vi "FTW-Inbox-Core-Configuration.vi"(5 "Inbox Configuration":string="{\n  \"MaxMessageSize\": 100000,\n  \"AdditionalServiceEndpoints\":\n  {\n    \"Primary\": \"tcp://127.0.0.1:*\",\n    \"RemoteClients\": \"ws://*:*\"\n  },\n  \"MessageRoutingRules\":\n  {\n    \"FTW-PoisonPill\":\n    {\n      \"Accept\": true,\n      \"Reject\": false\n    },\n    \"FTW-ActorStatus\":\n    {\n      \"Accept\": true,\n      \"Reject\": false,\n      \"BusyTimeout\": 100,\n      \"ResponseIncludesIdentity\": true,\n      \"ResponseIncludesTimestamp\": true,\n      \"ResponseIncludesRelativeTimer\": true\n    },\n    \"Default\":\n    {\n      \"Accept\": false,\n      \"Reject\": false,\n      \"BusyTimeout\": -1,\n      \"ResponseIncludesIdentity\": true,\n      \"ResponseIncludesTimestamp\": true,\n      \"ResponseIncludesRelativeTimer\": true\n    }\n  }\n}", 11 "error in":errorcluster) -> (4 "Message Routing Rules":T1[](array[typedef]) {"SendTimeout" format="%dmsec"; "BusyTimeout" format="%dmsec"}, 6 "Additional Endpoint Addresses":string[](array[string]), 8 "Receive Message Size Limit":i32=1000 format="%_4pbytes", 10 "AdditionalServiceEndpoints":string, 15 "error out":errorcluster)   [LabVIEW 2015]
uses:
  FTW-Inbox-Core-RoutingRule.ctl
  lib/FTW-KernelFilepath.vi
  error/FTW-ERR-ThrowError.vi
  json/core/FTW-JSON-Core-EncodingFlags.vi
  reflection/FTW-Reflection-Type.vi
  codegen/xnode/json/fetch/FTW-JSON-Core-GetFlattenedValue.vi
  error/FTW-ERR-NoErrorConstant.vi
  codegen/xnode/FTW-JSON-Fetch.xnode
panel:
  # "Inputs"
  # "Outputs"
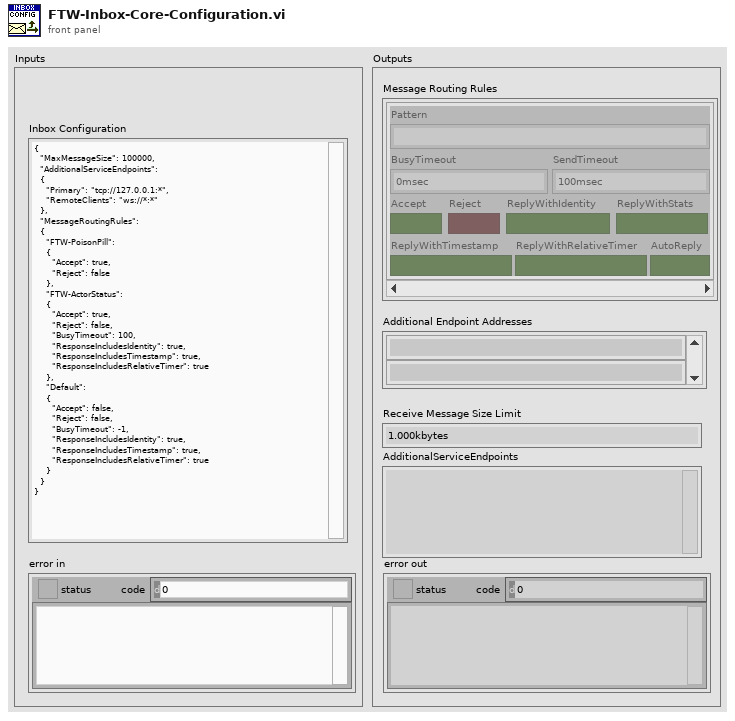
[diagram p1: front panel]
types:
  T1 = typedef "FTW-Inbox-Core-RoutingRule.ctl" = cluster{"Pattern":string, "BusyTimeout":i32, "SendTimeout":i32, "Accept":bool, "Reject":bool, "ReplyWithIdentity":bool, "ReplyWithStats":bool, "ReplyWithTimestamp":bool, "ReplyWithRelativeTimer":bool, "AutoReply":bool}
  T2 = cluster{"MaxMessageSize":i32, "MessageRoutingRules":string, "AdditionalServiceEndpoints":string, "MessageRoutingRules":cluster{"Default":cluster{"Pattern":string, "BusyTimeout":i32, "SendTimeout":i32, "Accept":bool, "Reject":bool, "ReplyWithIdentity":bool, "ReplyWithStatistics":bool, "ReplyWithTimestamp":bool, "ReplyWithRelativeTimer":bool, "AutoReply":bool}, "FTW-PoisonPill":cluster{"Pattern":string, "BusyTimeout":i32, "SendTimeout":i32, "Accept":bool, "Reject":bool, "ReplyWithIdentity":bool, "ReplyWithStatistics":bool, "ReplyWithTimestamp":bool, "ReplyWithRelativeTimer":bool, "AutoReply":bool}, "FTW-ActorStatus":cluster{"Pattern":string, "BusyTimeout":i32, "SendTimeout":i32, "Accept":bool, "Reject":bool, "ReplyWithIdentity":bool, "ReplyWithStatistics":bool, "ReplyWithTimestamp":bool, "ReplyWithRelativeTimer":bool, "AutoReply":bool}}}
  T3 = cluster{"Pattern":string, "BusyTimeout":i32, "SendTimeout":i32, "Accept":bool, "Reject":bool, "ReplyWithIdentity":bool, "ReplyWithStatistics":bool, "ReplyWithTimestamp":bool, "ReplyWithRelativeTimer":bool, "AutoReply":bool}
  T4 = typedef "FTW-Type-JSON.ctl" = refnum<data-value>
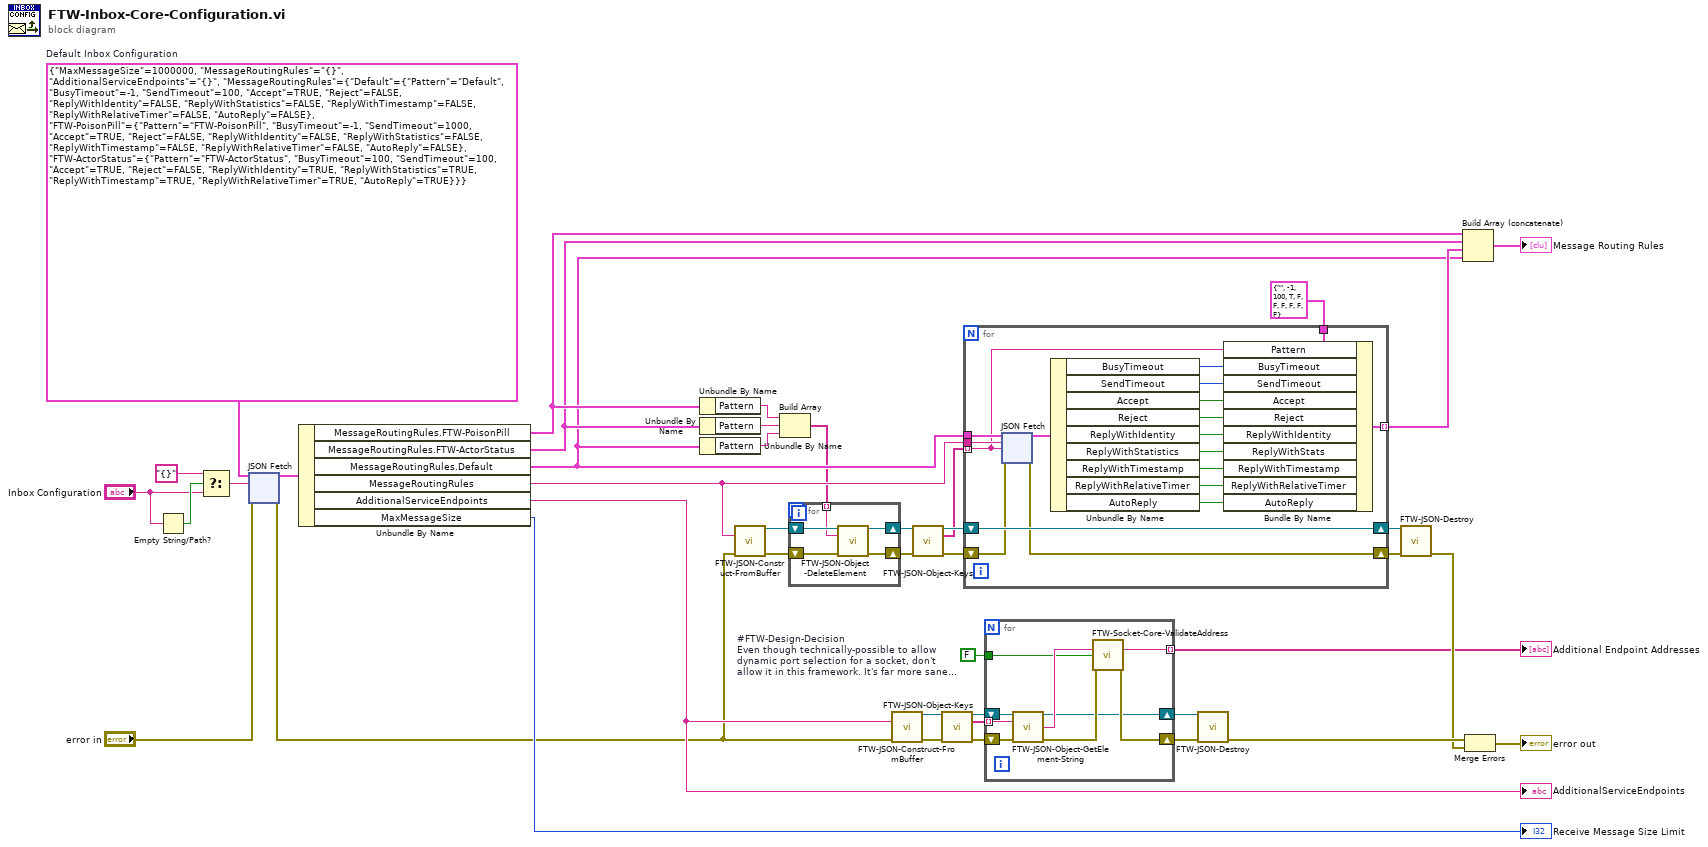
[diagram p0: block diagram]
diagram:
  w17 = FALSE  # #FTW-Design-Decision Even though technically-possible to allow dynamic port selection for a socket, don't allow it in this framework. It's far more sane to fix static addresses agreed upon by all nodes in the system.
  w5 = T2 {"MaxMessageSize"=1000000, "MessageRoutingRules"="{}", "AdditionalServiceEndpoints"="{}", "MessageRoutingRules"={"Default"={"Pattern"="Default", "BusyTimeout"=-1, "SendTimeout"=100, "Accept"=TRUE, "Reject"=FALSE, "ReplyWithIdentity"=FALSE, "ReplyWithStatistics"=FALSE, "ReplyWithTimestamp"=FALSE, "ReplyWithRelativeTimer"=FALSE, "AutoReply"=FALSE}, "FTW-PoisonPill"={"Pattern"="FTW-PoisonPill", "BusyTimeout"=-1, "SendTimeout"=1000, "Accept"=TRUE, "Reject"=FALSE, "ReplyWithIdentity"=FALSE, "ReplyWithStatistics"=FALSE, "ReplyWithTimestamp"=FALSE, "ReplyWithRelativeTimer"=FALSE, "AutoReply"=FALSE}, "FTW-ActorStatus"={"Pattern"="FTW-ActorStatus", "BusyTimeout"=100, "SendTimeout"=100, "Accept"=TRUE, "Reject"=FALSE, "ReplyWithIdentity"=TRUE, "ReplyWithStatistics"=TRUE, "ReplyWithTimestamp"=TRUE, "ReplyWithRelativeTimer"=TRUE, "AutoReply"=TRUE}}}  # Default Inbox Configuration
  n1 = Empty String/Path?(string/path="Inbox Configuration") -> (empty?=w8:bool)
  n2 = Select(t="{}", s=w8, f="Inbox Configuration") -> (s? t:f=w3:string)
  n3 = xnode "JSON Fetch"("Type and Defaults"=w5, "JSON String"=w3, "error in"="error in") -> ("Values"=w4:T2, "error out"=w1:errorcluster)  [unwired: 1 in]
  n4 = Unbundle By Name(w4) -> ("MessageRoutingRules.FTW-PoisonPill"=w15:T3, "MessageRoutingRules.FTW-ActorStatus"=w14:T3, "MessageRoutingRules.Default"=w13:T3, "MessageRoutingRules"=w16:string, "AdditionalServiceEndpoints"=w42:string, "MaxMessageSize"=→"Receive Message Size Limit":i32)
  "AdditionalServiceEndpoints" <- w42
  n5 = Unbundle By Name(w15) -> ("Pattern"=w12:string)
  n6 = Unbundle By Name(w14) -> ("Pattern"=w11:string)
  n7 = Unbundle By Name(w13) -> ("Pattern"=w10:string)
  n8 = call "FTW-JSON-Construct-FromBuffer.vi"("JSON String (UTF-8)"=w16, "error in"=w1) -> ("JSON"=w23:T4, "error out"=w21:errorcluster)  [unwired: 12 in]
  n9 = Build Array(w12, w11, w10) -> (w9:string[])
  n10 = for {
    shift-right: [w46] -> w22
    shift-left: w23 -> [w47]
    shift-right: [w44] -> w20
    shift-left: w21 -> [w45]
    tunnel: w9 -> [w43] mode=indexing
    n11 = call "FTW-JSON-Object-DeleteElement.vi"("JSON"=w47, "Key"=w43, "error in"=w45) -> ("JSON out"=w46:T4, "error out"=w44:errorcluster)  [unwired: 10 in, 1 out]
  }
  n12 = call "FTW-JSON-Construct-FromBuffer.vi"("JSON String (UTF-8)"=w42, "error in"=w1) -> ("JSON"=w36:T4, "error out"=w35:errorcluster)  [unwired: 12 in]
  n13 = call "FTW-JSON-Object-Keys.vi"("JSON"=w22, "error in"=w20) -> ("JSON out"=w31:T4, "Keys"=w30:string[], "error out"=w32:errorcluster)  [unwired: 11 in]
  n14 = call "FTW-JSON-Object-Keys.vi"("JSON"=w36, "error in"=w35) -> ("JSON out"=w40:T4, "Keys"=w41:string[], "error out"=w39:errorcluster)  [unwired: 11 in]
  n15 = for {
    shift-right: [w49] -> w34
    shift-left: w32 -> [w50]
    tunnel: w30 -> [w48] mode=indexing
    shift-right: [w65] -> w33
    shift-left: w31 -> [w65]
    tunnel: w13 -> [w53]
    tunnel: w16 -> [w51]
    tunnel: [w63] -> w18 mode=indexing
    tunnel: T1 {"Pattern"="", "BusyTimeout"=-1, "SendTimeout"=100, "Accept"=TRUE, "Reject"=FALSE, "ReplyWithIdentity"=FALSE, "ReplyWithStats"=FALSE, "ReplyWithTimestamp"=FALSE, "ReplyWithRelativeTimer"=FALSE, "AutoReply"=FALSE} ("Routing Rule") -> [w64]
    n16 = xnode "JSON Fetch"("Type and Defaults"=w53, "JSON String"=w51, "Element Path"=w48, "error in"=w50) -> ("Values"=w52:T3, "error out"=w49:errorcluster)
    n17 = Unbundle By Name(w52) -> ("BusyTimeout"=w62:i32, "SendTimeout"=w61:i32, "Accept"=w60:bool, "Reject"=w59:bool, "ReplyWithIdentity"=w58:bool, "ReplyWithStatistics"=w57:bool, "ReplyWithTimestamp"=w56:bool, "ReplyWithRelativeTimer"=w55:bool, "AutoReply"=w54:bool)
    n18 = Bundle By Name(cluster=w64, "Pattern"=w48, "BusyTimeout"=w62, "SendTimeout"=w61, "Accept"=w60, "Reject"=w59, "ReplyWithIdentity"=w58, "ReplyWithStats"=w57, "ReplyWithTimestamp"=w56, "ReplyWithRelativeTimer"=w55, "AutoReply"=w54) -> (w63:T1)
  }
  n19 = for {
    tunnel: [w139] -> w24 mode=indexing
    shift-right: [w140] -> w37
    shift-left: w39 -> [w135]
    tunnel: w41 -> [w137] mode=indexing
    shift-right: [w133] -> w38
    shift-left: w40 -> [w138]
    tunnel: w17 -> [w132]
    n20 = call "FTW-JSON-Object-GetElement-String.vi"("JSON"=w138, "Key"=w137, "error in"=w135) -> ("JSON out"=w133:T4, "Value"=w136:string, "error out"=w134:errorcluster)  [unwired: 9 in, 1 out]
    n21 = call "FTW-Socket-Core-ValidateAddress.vi"("Address"=w136, "Allow wildcard replacement?"=w132, "error in"=w134) -> ("Sanitized Address"=w139:string, "error out"=w140:errorcluster)  [unwired: 10 in, 1 out]
  }
  "Additional Endpoint Addresses" <- w24
  n22 = call "FTW-JSON-Destroy.vi"("JSON"=w38, "error in"=w37) -> ("error out"=w29:errorcluster)  [unwired: 13 in]
  n23 = call "FTW-JSON-Destroy.vi"("JSON"=w33, "error in"=w34) -> ("error out"=w27:errorcluster)  [unwired: 13 in]
  n24 = Build Array (concatenate)(w15, w14, w18, w13) -> (→"Message Routing Rules":T1[])
  n25 = Merge Errors(w29, w27) -> (→"error out":errorcluster)
